vi "TW Call gRPC Scripting.vi"(8 "error in":errorcluster, 10 "gRPC Service Name":string, 11 "proto File Path":path) -> (0 "error out":errorcluster)   [LabVIEW 2021, in "Plugin Generator.lvlib"]
uses:
  Plugin Generator.lvlib
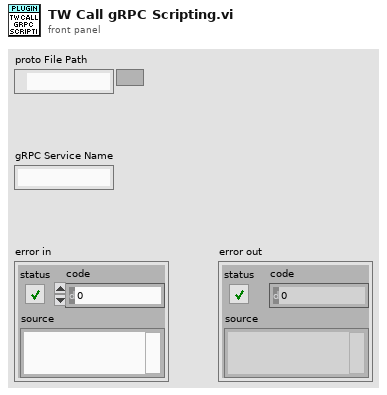
[diagram p1: front panel]
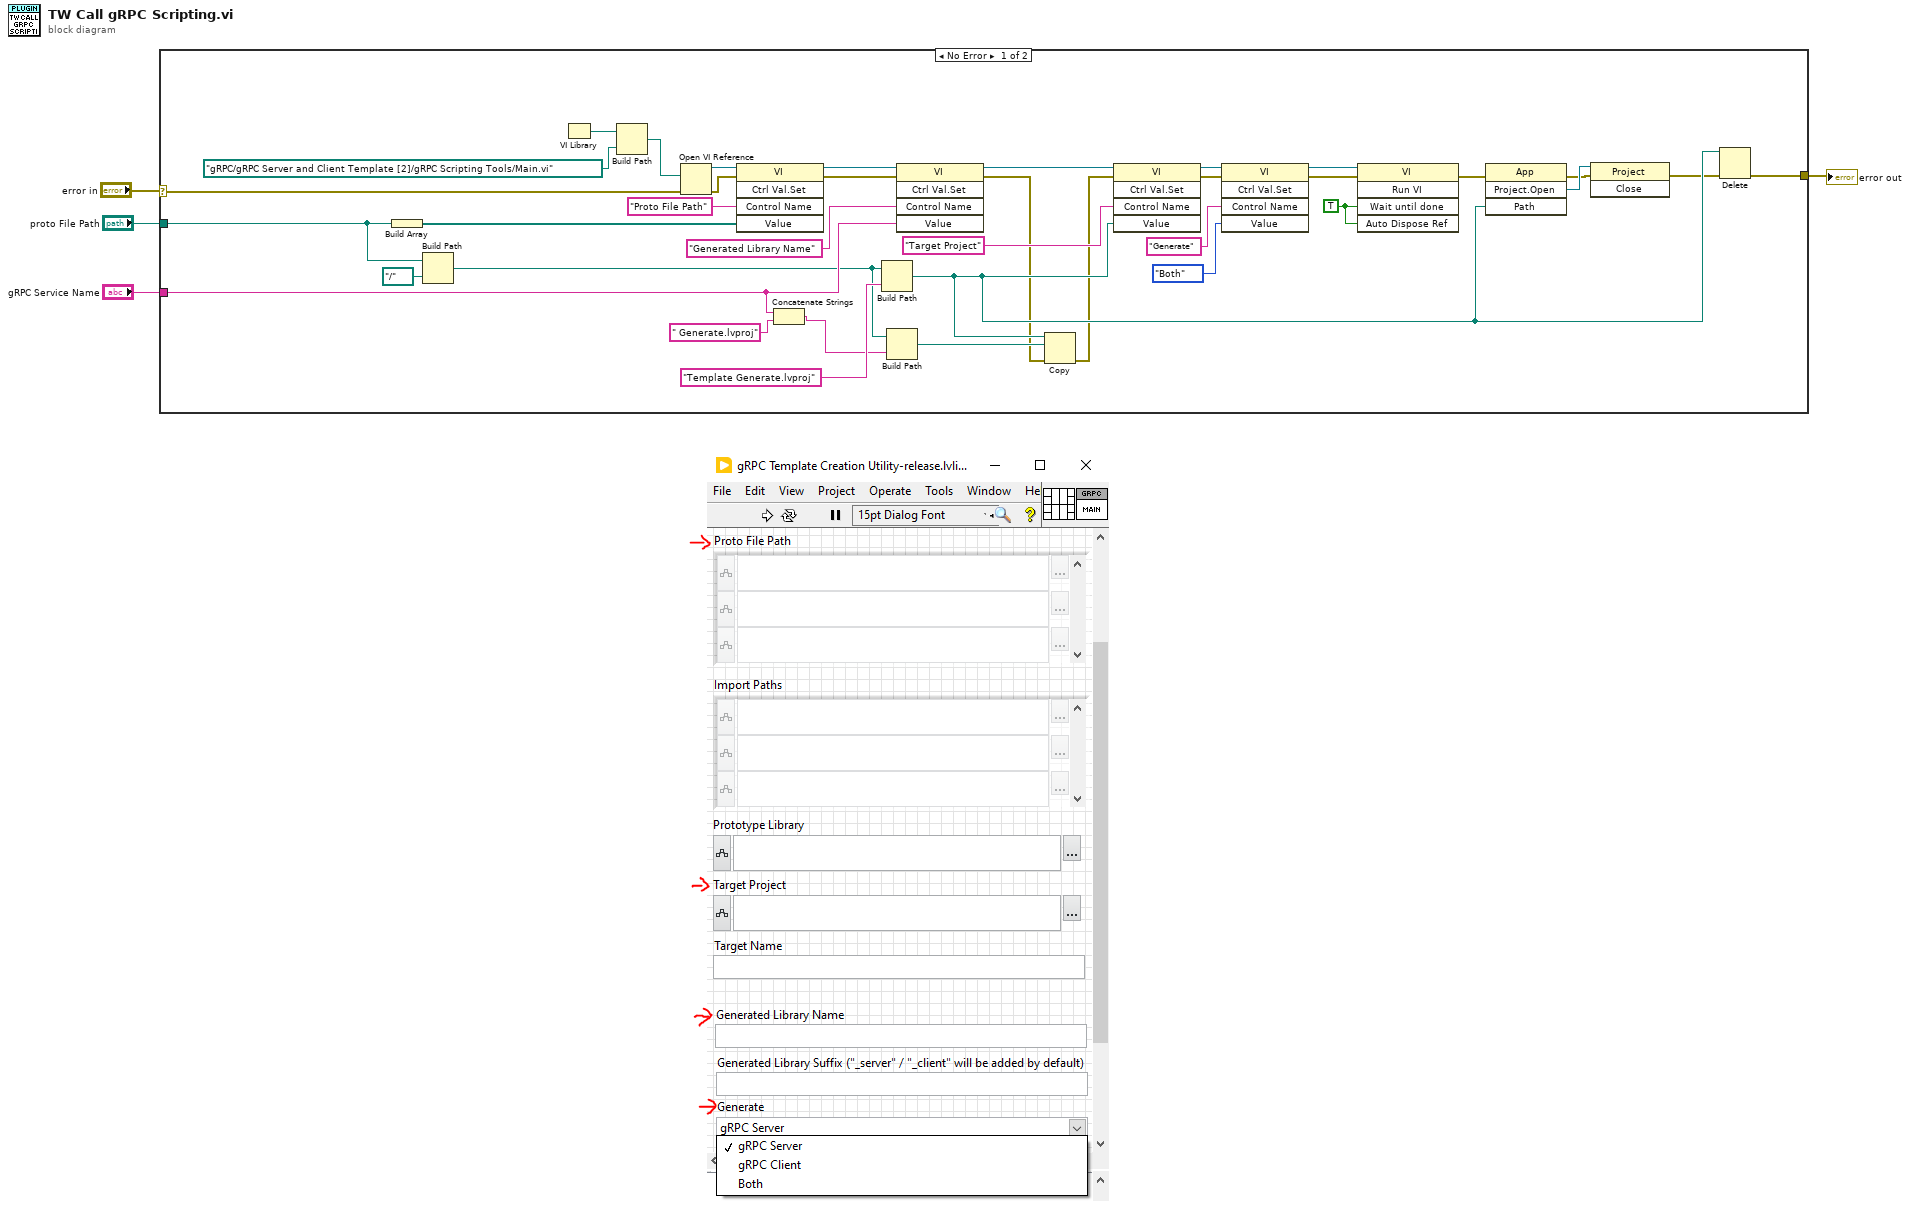
[diagram p0: block diagram]
diagram:
  n1 = case shown="No Error" "error in" {
    selector: "error in" -> [w5 w41]
    tunnel: [w10 w41] -> w4
    tunnel: "gRPC Service Name" -> [w17 _]
    tunnel: "proto File Path" -> [w16 _]
    frame No Error {
      w18 = TRUE ("Wait Until Done")
      n2 = Build Array(w16) -> (w23:path[])
      n3 = Build Path(base path=w16, name or relative path=path "../..") -> (appended path=w13:path)
      n4 = VI Library() -> (path=w40:path)
      n5 = Build Path(base path=w40, name or relative path=path "gRPC/gRPC Server and Client Template [2]/gRPC Scripting Tools/Main.vi") -> (appended path=w38:path)
      n6 = Open VI Reference(vi path=w38, error in (no error)=w5) -> (vi reference=w25:refnum<vi>, error out=w24:errorcluster)  [unwired: 4 in]
      n7 = invoke class="VI" method="Ctrl Val.Set"(reference=w25, error in=w24, "Control Name"="Proto File Path", "Value"=w23) -> (reference out=w36:refnum<vi>, error out=w35:errorcluster)  [unwired: 1 in, 3 out]
      n8 = Concatenate Strings(w17, " Generate.lvproj" ("string")) -> (w12:string)
      n9 = Build Path(base path=w13, name or relative path="Template Generate.lvproj" ("string")) -> (appended path=w9:path)
      n10 = Build Path(base path=w13, name or relative path=w12) -> (appended path=w11:path)
      n11 = invoke class="VI" method="Ctrl Val.Set"(reference=w36, error in=w35, "Control Name"="Generated Library Name", "Value"=w17) -> (reference out=w33:refnum<vi>, error out=w8:errorcluster)  [unwired: 1 in, 3 out]
      n12 = Copy(8:w8, 10:w11, 11:w9) -> (0:w7:errorcluster)  [unwired: 2 in, 2 out]
      n13 = invoke class="VI" method="Ctrl Val.Set"(reference=w33, error in=w7, "Control Name"="Target Project", "Value"=w9) -> (reference out=w31:refnum<vi>, error out=w30:errorcluster)  [unwired: 1 in, 3 out]
      n14 = invoke class="VI" method="Ctrl Val.Set"(reference=w31, error in=w30, "Control Name"="Generate", "Value"=enum16{"gRPC Server", "gRPC Client", "Both"}."Both" ("Generate")) -> (reference out=w27:refnum<vi>, error out=w26:errorcluster)  [unwired: 1 in, 3 out]
      n15 = invoke class="VI" method="Run VI"(reference=w27, error in=w26, "Wait until done"=w18, "Auto Dispose Ref"=w18) -> (error out=w19:errorcluster)  [unwired: 1 in, 4 out]
      n16 = invoke class="App" method="Project.Open"(error in=w19, "Path"=w9) -> (error out=w20:errorcluster, "Project:Open"=w21:refnum<vi>)  [unwired: 2 in, 2 out]
      n17 = invoke class="Project" method="Close"(reference=w21, error in=w20) -> (error out=w6:errorcluster)  [unwired: 1 in, 2 out]
      n18 = Delete(path (use dialog)=w9, error in=w6) -> (error out=w10:errorcluster)  [unwired: 3 in, 2 out]
    }
    frame Error {
    }
  }
  "error out" <- w4
